vi "Condition Private Data.vi"(8 "error in":errorcluster, 9 "Private Data Cluster":refnum<vi>, 10 "Private Data Control":refnum<vi>) -> (0 "error out":errorcluster)   [LabVIEW 2025, in "_Rescript.lvlib" / "_Rescript.lvclass"]
uses:
  _Rescript.lvclass
  _Rescript.lvclass/_Rescript.ctl
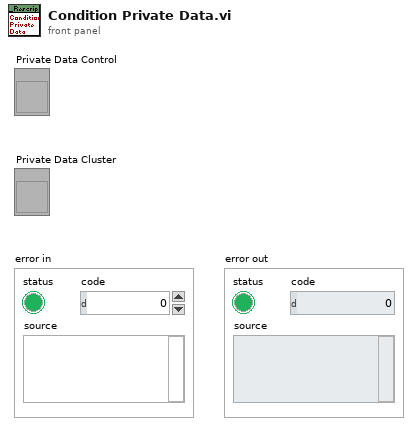
[diagram p1: front panel]
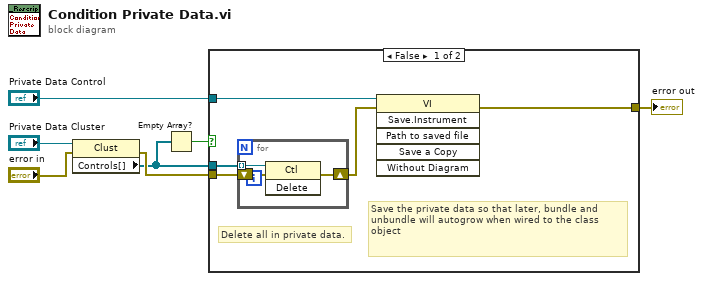
[diagram p0: block diagram]
diagram:
  n1 = property class="Clust"(reference="Private Data Cluster", error in="error in") -> (error out=w7:errorcluster, "Controls[]"=w4:refnum<vi>[])  [unwired: 1 out]
  n2 = Empty Array?(array=w4) -> (empty?=w3:bool)
  n3 = case shown="False" w3 {
    tunnel: w4 -> [w12 _]
    tunnel: w7 -> [w11 w16]
    tunnel: [w9 w16] -> w2
    tunnel: "Private Data Control" -> [w8 _]
    frame False {
      # "Save the private data so that later, bundle and unbundle will autogrow when wired to the class object"
      # "Delete all in private data."
      n4 = for {
        tunnel: w12 -> [w15] mode=indexing
        shift-right: [w13] -> w10
        shift-left: w11 -> [w14]
        n5 = invoke class="Ctl" method="Delete"(reference=w15, error in=w14) -> (error out=w13:errorcluster)  [unwired: 1 in, 2 out]
      }
      n6 = invoke class="VI" method="Save.Instrument"(reference=w8, error in=w10) -> (error out=w9:errorcluster)  [unwired: 4 in, 5 out]
    }
    frame True {
    }
  }
  "error out" <- w2
